vi "createTrack.vi"() -> (0 "Course":T1(array[cluster]), 2 "verticalCourse":cluster{"X":sgl, "Y":sgl}[](array[cluster])=[{"X"=-400.0, "Y"=600.0}, {"X"=-200.0, "Y"=600.0}, {"X"=0.0, "Y"=600.0}, {"X"=200.0, "Y"=600.0}, {"X"=400.0, "Y"=600.0}], 3 "hoizontalCourse":cluster{"X":sgl, "Y":sgl}[](array[cluster])=[{"X"=-400.0, "Y"=600.0}, {"X"=-200.0, "Y"=600.0}, {"X"=0.0, "Y"=600.0}, {"X"=200.0, "Y"=600.0}, {"X"=400.0, "Y"=600.0}])   [LabVIEW 2015]
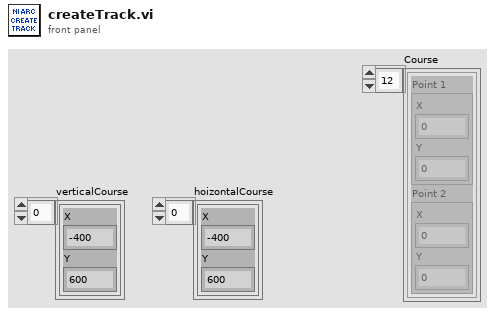
[diagram p1: front panel]
types:
  T1 = cluster{"Point 1":cluster{"X":sgl, "Y":sgl}, "Point 2":cluster{"X":sgl, "Y":sgl}}[]
  T2 = cluster{"Point 1":cluster{"X":sgl, "Y":sgl}, "Point 2":cluster{"X":sgl, "Y":sgl}}
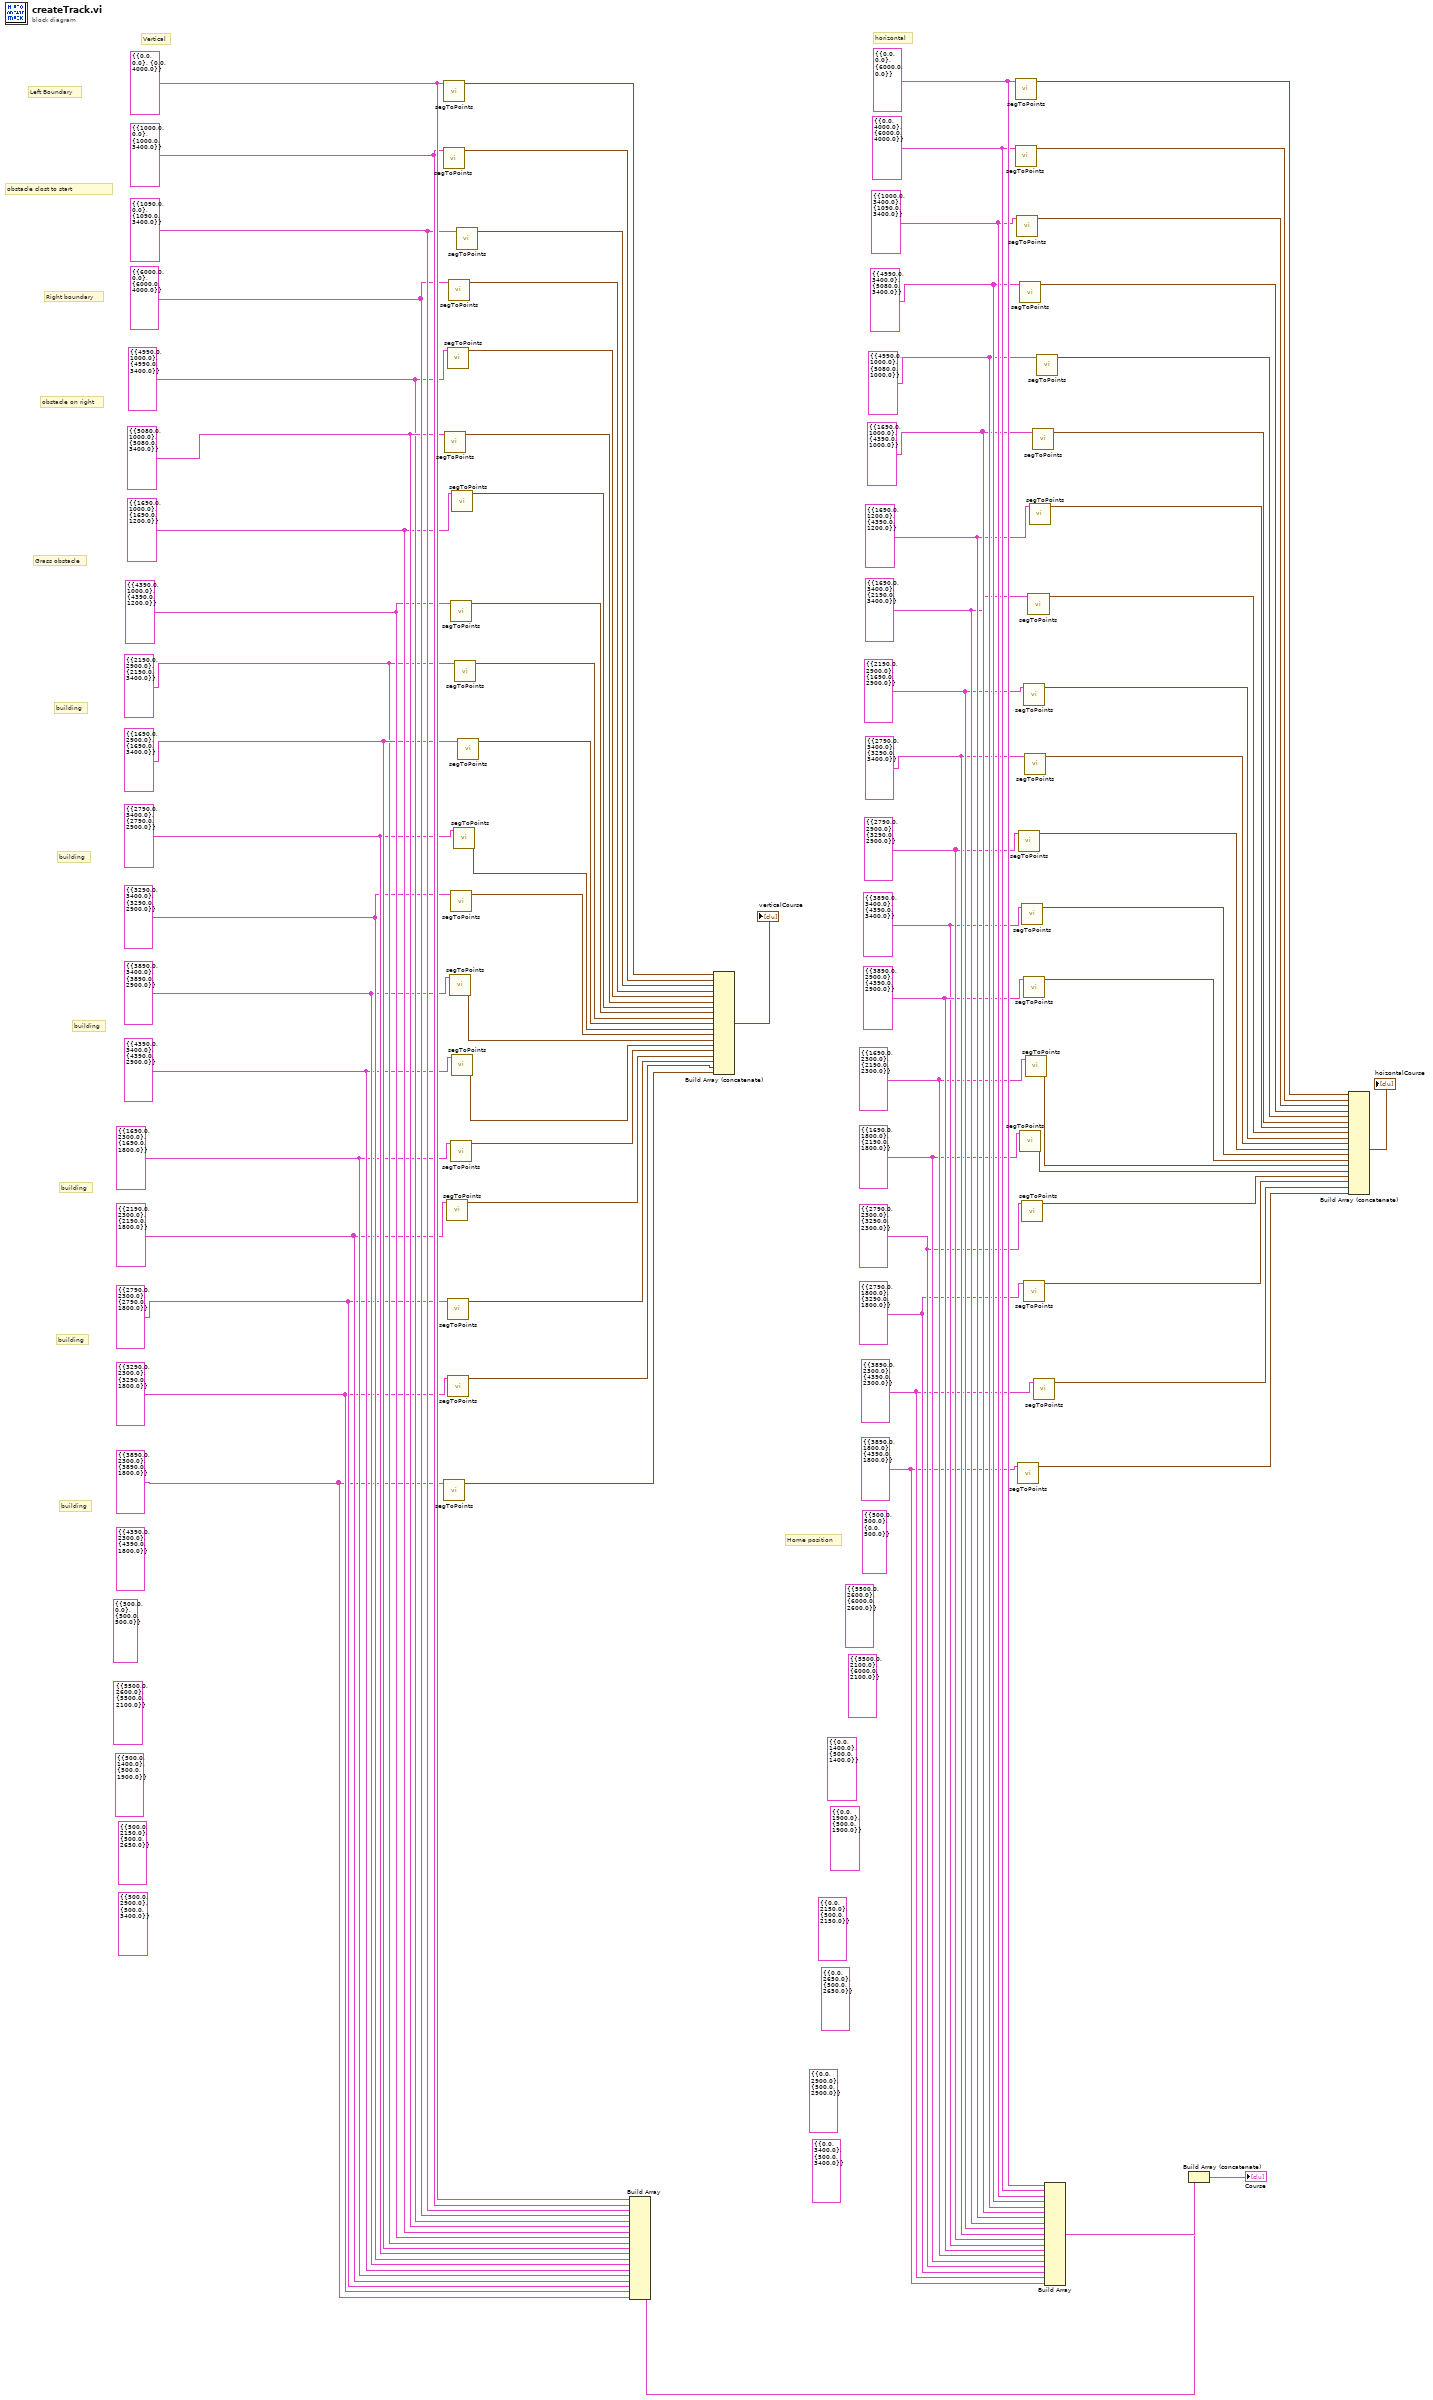
[diagram p0: block diagram]
diagram:
  (unwired) T2 {"Point 1"={"X"=0.0, "Y"=3400.0}, "Point 2"={"X"=500.0, "Y"=3400.0}} ("Line Segment")
  (unwired) T2 {"Point 1"={"X"=0.0, "Y"=2900.0}, "Point 2"={"X"=500.0, "Y"=2900.0}} ("Line Segment")
  (unwired) T2 {"Point 1"={"X"=0.0, "Y"=2650.0}, "Point 2"={"X"=500.0, "Y"=2650.0}} ("Line Segment")
  (unwired) T2 {"Point 1"={"X"=0.0, "Y"=2150.0}, "Point 2"={"X"=500.0, "Y"=2150.0}} ("Line Segment")
  (unwired) T2 {"Point 1"={"X"=0.0, "Y"=1900.0}, "Point 2"={"X"=500.0, "Y"=1900.0}} ("Line Segment")
  (unwired) T2 {"Point 1"={"X"=0.0, "Y"=1400.0}, "Point 2"={"X"=500.0, "Y"=1400.0}} ("Line Segment")
  (unwired) T2 {"Point 1"={"X"=500.0, "Y"=2900.0}, "Point 2"={"X"=500.0, "Y"=3400.0}} ("Line Segment")
  (unwired) T2 {"Point 1"={"X"=500.0, "Y"=2150.0}, "Point 2"={"X"=500.0, "Y"=2650.0}} ("Line Segment")
  (unwired) T2 {"Point 1"={"X"=500.0, "Y"=1400.0}, "Point 2"={"X"=500.0, "Y"=1900.0}} ("Line Segment")
  (unwired) T2 {"Point 1"={"X"=5500.0, "Y"=2600.0}, "Point 2"={"X"=5500.0, "Y"=2100.0}} ("Line Segment")
  (unwired) T2 {"Point 1"={"X"=5500.0, "Y"=2100.0}, "Point 2"={"X"=6000.0, "Y"=2100.0}} ("Line Segment")
  (unwired) T2 {"Point 1"={"X"=5500.0, "Y"=2600.0}, "Point 2"={"X"=6000.0, "Y"=2600.0}} ("Line Segment")
  (unwired) T2 {"Point 1"={"X"=500.0, "Y"=500.0}, "Point 2"={"X"=0.0, "Y"=500.0}} ("Line Segment")
  (unwired) T2 {"Point 1"={"X"=500.0, "Y"=0.0}, "Point 2"={"X"=500.0, "Y"=500.0}} ("Line Segment")
  w10 = T2 {"Point 1"={"X"=3890.0, "Y"=1800.0}, "Point 2"={"X"=4390.0, "Y"=1800.0}} ("Line Segment")
  w11 = T2 {"Point 1"={"X"=3890.0, "Y"=2300.0}, "Point 2"={"X"=4390.0, "Y"=2300.0}} ("Line Segment")
  (unwired) T2 {"Point 1"={"X"=4390.0, "Y"=2300.0}, "Point 2"={"X"=4390.0, "Y"=1800.0}} ("Line Segment")
  w5 = T2 {"Point 1"={"X"=3890.0, "Y"=2300.0}, "Point 2"={"X"=3890.0, "Y"=1800.0}} ("Line Segment")
  w15 = T2 {"Point 1"={"X"=2790.0, "Y"=1800.0}, "Point 2"={"X"=3290.0, "Y"=1800.0}} ("Line Segment")
  w16 = T2 {"Point 1"={"X"=2790.0, "Y"=2300.0}, "Point 2"={"X"=3290.0, "Y"=2300.0}} ("Line Segment")
  w6 = T2 {"Point 1"={"X"=3290.0, "Y"=2300.0}, "Point 2"={"X"=3290.0, "Y"=1800.0}} ("Line Segment")
  w17 = T2 {"Point 1"={"X"=2790.0, "Y"=2300.0}, "Point 2"={"X"=2790.0, "Y"=1800.0}} ("Line Segment")
  w23 = T2 {"Point 1"={"X"=1690.0, "Y"=1800.0}, "Point 2"={"X"=2190.0, "Y"=1800.0}} ("Line Segment")
  w24 = T2 {"Point 1"={"X"=1690.0, "Y"=2300.0}, "Point 2"={"X"=2190.0, "Y"=2300.0}} ("Line Segment")
  w21 = T2 {"Point 1"={"X"=2190.0, "Y"=2300.0}, "Point 2"={"X"=2190.0, "Y"=1800.0}} ("Line Segment")
  w22 = T2 {"Point 1"={"X"=1690.0, "Y"=2300.0}, "Point 2"={"X"=1690.0, "Y"=1800.0}} ("Line Segment")
  w31 = T2 {"Point 1"={"X"=3890.0, "Y"=2900.0}, "Point 2"={"X"=4390.0, "Y"=2900.0}} ("Line Segment")
  w25 = T2 {"Point 1"={"X"=3890.0, "Y"=3400.0}, "Point 2"={"X"=4390.0, "Y"=3400.0}} ("Line Segment")
  w29 = T2 {"Point 1"={"X"=4390.0, "Y"=3400.0}, "Point 2"={"X"=4390.0, "Y"=2900.0}} ("Line Segment")
  w30 = T2 {"Point 1"={"X"=3890.0, "Y"=3400.0}, "Point 2"={"X"=3890.0, "Y"=2900.0}} ("Line Segment")
  w38 = T2 {"Point 1"={"X"=3290.0, "Y"=3400.0}, "Point 2"={"X"=3290.0, "Y"=2900.0}} ("Line Segment")
  w39 = T2 {"Point 1"={"X"=2790.0, "Y"=3400.0}, "Point 2"={"X"=2790.0, "Y"=2900.0}} ("Line Segment")
  w40 = T2 {"Point 1"={"X"=2790.0, "Y"=2900.0}, "Point 2"={"X"=3290.0, "Y"=2900.0}} ("Line Segment")
  w41 = T2 {"Point 1"={"X"=2790.0, "Y"=3400.0}, "Point 2"={"X"=3290.0, "Y"=3400.0}} ("Line Segment")
  w44 = T2 {"Point 1"={"X"=2190.0, "Y"=2900.0}, "Point 2"={"X"=1690.0, "Y"=2900.0}} ("Line Segment")
  w45 = T2 {"Point 1"={"X"=1690.0, "Y"=3400.0}, "Point 2"={"X"=2190.0, "Y"=3400.0}} ("Line Segment")
  w52 = T2 {"Point 1"={"X"=1690.0, "Y"=2900.0}, "Point 2"={"X"=1690.0, "Y"=3400.0}} ("Line Segment")
  w43 = T2 {"Point 1"={"X"=2190.0, "Y"=2900.0}, "Point 2"={"X"=2190.0, "Y"=3400.0}} ("Line Segment")
  w53 = T2 {"Point 1"={"X"=4390.0, "Y"=1000.0}, "Point 2"={"X"=4390.0, "Y"=1200.0}} ("Line Segment")
  w54 = T2 {"Point 1"={"X"=1690.0, "Y"=1000.0}, "Point 2"={"X"=1690.0, "Y"=1200.0}} ("Line Segment")
  w55 = T2 {"Point 1"={"X"=1690.0, "Y"=1200.0}, "Point 2"={"X"=4390.0, "Y"=1200.0}} ("Line Segment")
  w56 = T2 {"Point 1"={"X"=1690.0, "Y"=1000.0}, "Point 2"={"X"=4390.0, "Y"=1000.0}} ("Line Segment")
  w61 = T2 {"Point 1"={"X"=5080.0, "Y"=1000.0}, "Point 2"={"X"=5080.0, "Y"=3400.0}} ("Line Segment")
  w60 = T2 {"Point 1"={"X"=4990.0, "Y"=1000.0}, "Point 2"={"X"=4990.0, "Y"=3400.0}} ("Line Segment")
  w62 = T2 {"Point 1"={"X"=4990.0, "Y"=1000.0}, "Point 2"={"X"=5080.0, "Y"=1000.0}} ("Line Segment")
  w65 = T2 {"Point 1"={"X"=4990.0, "Y"=3400.0}, "Point 2"={"X"=5080.0, "Y"=3400.0}} ("Line Segment")
  w67 = T2 {"Point 1"={"X"=6000.0, "Y"=0.0}, "Point 2"={"X"=6000.0, "Y"=4000.0}} ("Line Segment")
  w69 = T2 {"Point 1"={"X"=1000.0, "Y"=3400.0}, "Point 2"={"X"=1090.0, "Y"=3400.0}} ("Line Segment")
  w70 = T2 {"Point 1"={"X"=1090.0, "Y"=0.0}, "Point 2"={"X"=1090.0, "Y"=3400.0}} ("Line Segment")
  w75 = T2 {"Point 1"={"X"=0.0, "Y"=4000.0}, "Point 2"={"X"=6000.0, "Y"=4000.0}} ("Line Segment")
  w76 = T2 {"Point 1"={"X"=0.0, "Y"=0.0}, "Point 2"={"X"=6000.0, "Y"=0.0}} ("Line Segment")
  w73 = T2 {"Point 1"={"X"=1000.0, "Y"=0.0}, "Point 2"={"X"=1000.0, "Y"=3400.0}} ("Line Segment")
  w74 = T2 {"Point 1"={"X"=0.0, "Y"=0.0}, "Point 2"={"X"=0.0, "Y"=4000.0}} ("Line Segment")
  # "Home position"
  # "Left Boundary"
  # "obstacle clost to start"
  # "Right boundary"
  # "obstacle on right"
  # "Grass obstacle"
  # "building"
  # "building"
  # "building"
  # "building"
  # "building"
  # "building"
  # "horizontal"
  # "Vertical"
  n1 = call "segToPoints.vi"("Line Segment"=w73) -> ("points"=w80:cluster{"X":sgl, "Y":sgl}[])  [unwired: 10 in]
  n2 = call "segToPoints.vi"("Line Segment"=w74) -> ("points"=w81:cluster{"X":sgl, "Y":sgl}[])  [unwired: 10 in]
  n3 = call "segToPoints.vi"("Line Segment"=w5) -> ("points"=w9:cluster{"X":sgl, "Y":sgl}[])  [unwired: 10 in]
  n4 = call "segToPoints.vi"("Line Segment"=w61) -> ("points"=w63:cluster{"X":sgl, "Y":sgl}[])  [unwired: 10 in]
  n5 = call "segToPoints.vi"("Line Segment"=w21) -> ("points"=w27:cluster{"X":sgl, "Y":sgl}[])  [unwired: 10 in]
  n6 = call "segToPoints.vi"("Line Segment"=w60) -> ("points"=w64:cluster{"X":sgl, "Y":sgl}[])  [unwired: 10 in]
  n7 = call "segToPoints.vi"("Line Segment"=w17) -> ("points"=w19:cluster{"X":sgl, "Y":sgl}[])  [unwired: 10 in]
  n8 = call "segToPoints.vi"("Line Segment"=w6) -> ("points"=w18:cluster{"X":sgl, "Y":sgl}[])  [unwired: 10 in]
  n9 = call "segToPoints.vi"("Line Segment"=w67) -> ("points"=w49:cluster{"X":sgl, "Y":sgl}[])  [unwired: 10 in]
  n10 = call "segToPoints.vi"("Line Segment"=w30) -> ("points"=w35:cluster{"X":sgl, "Y":sgl}[])  [unwired: 10 in]
  n11 = call "segToPoints.vi"("Line Segment"=w53) -> ("points"=w59:cluster{"X":sgl, "Y":sgl}[])  [unwired: 10 in]
  n12 = call "segToPoints.vi"("Line Segment"=w38) -> ("points"=w42:cluster{"X":sgl, "Y":sgl}[])  [unwired: 10 in]
  n13 = call "segToPoints.vi"("Line Segment"=w22) -> ("points"=w28:cluster{"X":sgl, "Y":sgl}[])  [unwired: 10 in]
  n14 = call "segToPoints.vi"("Line Segment"=w29) -> ("points"=w34:cluster{"X":sgl, "Y":sgl}[])  [unwired: 10 in]
  n15 = call "segToPoints.vi"("Line Segment"=w54) -> ("points"=w58:cluster{"X":sgl, "Y":sgl}[])  [unwired: 10 in]
  n16 = call "segToPoints.vi"("Line Segment"=w39) -> ("points"=w20:cluster{"X":sgl, "Y":sgl}[])  [unwired: 10 in]
  n17 = call "segToPoints.vi"("Line Segment"=w43) -> ("points"=w51:cluster{"X":sgl, "Y":sgl}[])  [unwired: 10 in]
  n18 = call "segToPoints.vi"("Line Segment"=w70) -> ("points"=w50:cluster{"X":sgl, "Y":sgl}[])  [unwired: 10 in]
  n19 = call "segToPoints.vi"("Line Segment"=w52) -> ("points"=w48:cluster{"X":sgl, "Y":sgl}[])  [unwired: 10 in]
  n20 = Build Array(w74, w73, w70, w67, w60, w61, w54, w53, w43, w52, w39, w38, w30, w29, w22, w21, w17, w6, w5) -> (w1:T1)
  n21 = Build Array (concatenate)(w81, w80, w50, w49, w64, w63, w58, w59, w51, w48, w20, w42, w35, w34, w28, w27, w19, w18, w9) -> (→"verticalCourse":cluster{"X":sgl, "Y":sgl}[])
  n22 = call "segToPoints.vi"("Line Segment"=w75) -> ("points"=w79:cluster{"X":sgl, "Y":sgl}[])  [unwired: 10 in]
  n23 = call "segToPoints.vi"("Line Segment"=w76) -> ("points"=w2:cluster{"X":sgl, "Y":sgl}[])  [unwired: 10 in]
  n24 = call "segToPoints.vi"("Line Segment"=w69) -> ("points"=w68:cluster{"X":sgl, "Y":sgl}[])  [unwired: 10 in]
  n25 = call "segToPoints.vi"("Line Segment"=w10) -> ("points"=w7:cluster{"X":sgl, "Y":sgl}[])  [unwired: 10 in]
  n26 = call "segToPoints.vi"("Line Segment"=w40) -> ("points"=w36:cluster{"X":sgl, "Y":sgl}[])  [unwired: 10 in]
  n27 = call "segToPoints.vi"("Line Segment"=w65) -> ("points"=w66:cluster{"X":sgl, "Y":sgl}[])  [unwired: 10 in]
  n28 = call "segToPoints.vi"("Line Segment"=w23) -> ("points"=w4:cluster{"X":sgl, "Y":sgl}[])  [unwired: 10 in]
  n29 = call "segToPoints.vi"("Line Segment"=w25) -> ("points"=w33:cluster{"X":sgl, "Y":sgl}[])  [unwired: 10 in]
  n30 = call "segToPoints.vi"("Line Segment"=w16) -> ("points"=w13:cluster{"X":sgl, "Y":sgl}[])  [unwired: 10 in]
  n31 = call "segToPoints.vi"("Line Segment"=w31) -> ("points"=w32:cluster{"X":sgl, "Y":sgl}[])  [unwired: 10 in]
  n32 = call "segToPoints.vi"("Line Segment"=w15) -> ("points"=w12:cluster{"X":sgl, "Y":sgl}[])  [unwired: 10 in]
  n33 = call "segToPoints.vi"("Line Segment"=w44) -> ("points"=w46:cluster{"X":sgl, "Y":sgl}[])  [unwired: 10 in]
  n34 = call "segToPoints.vi"("Line Segment"=w41) -> ("points"=w37:cluster{"X":sgl, "Y":sgl}[])  [unwired: 10 in]
  n35 = call "segToPoints.vi"("Line Segment"=w24) -> ("points"=w26:cluster{"X":sgl, "Y":sgl}[])  [unwired: 10 in]
  n36 = call "segToPoints.vi"("Line Segment"=w45) -> ("points"=w47:cluster{"X":sgl, "Y":sgl}[])  [unwired: 10 in]
  n37 = call "segToPoints.vi"("Line Segment"=w55) -> ("points"=w3:cluster{"X":sgl, "Y":sgl}[])  [unwired: 10 in]
  n38 = call "segToPoints.vi"("Line Segment"=w56) -> ("points"=w57:cluster{"X":sgl, "Y":sgl}[])  [unwired: 10 in]
  n39 = call "segToPoints.vi"("Line Segment"=w11) -> ("points"=w8:cluster{"X":sgl, "Y":sgl}[])  [unwired: 10 in]
  n40 = call "segToPoints.vi"("Line Segment"=w62) -> ("points"=w14:cluster{"X":sgl, "Y":sgl}[])  [unwired: 10 in]
  n41 = Build Array(w76, w75, w69, w65, w62, w56, w55, w45, w44, w41, w40, w25, w31, w24, w23, w16, w15, w11, w10) -> (w72:T1)
  n42 = Build Array (concatenate)(w72, w1) -> (→"Course":T1)
  n43 = Build Array (concatenate)(w2, w79, w68, w66, w14, w57, w3, w47, w46, w37, w36, w33, w32, w26, w4, w13, w12, w8, w7) -> (→"hoizontalCourse":cluster{"X":sgl, "Y":sgl}[])
